vi "Global_Izleme.vi"() -> ()   [LabVIEW 2014]
uses:
  CustomControls/TSE_Status.ctl
  CustomControls/Program_States.ctl
  SharedVariables/TSE_Variables.vi
panel:
  in  "stop":bool
  out "TSE Status":T1={"Return Code"=0, "Message"="", "error in (no error)"={"status"=FALSE, "code"=0, "source"=""}, "Program State"=enum."Ön Yükleme Tamam", "Test A. Suresi"=0}
  out "GPIB_Interface_No":string
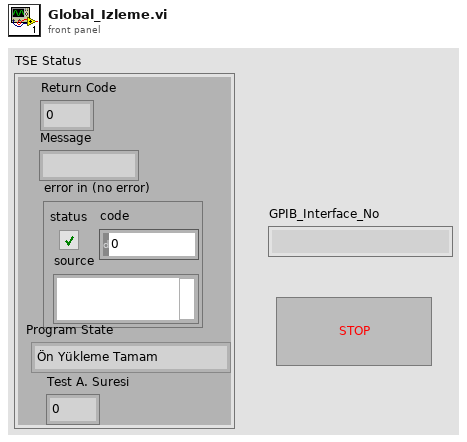
[diagram p1: front panel]
types:
  T1 = typedef "TSE_Status.ctl" = cluster{"Return Code":i32, "Message":string, "error in (no error)":errorcluster, "Program State":T2, "Test A. Suresi":u32}
  T2 = typedef "Program_States.ctl" = enum16{"Ön Yükleme", "TSE Baslat", "Kalibratöre Baglan", "Kalibratörü Baslat", "Ön Yükleme Tamam", "Frekans Testi", "Gerilim Testi", "Akim Testi", "Aktif Guc Testi", "Reaktif Guc Testi", "AC Akim Harmonik Testi", "AC Gerilim Harmonik Testi", "Flicker Testi", "Rapor Cikarma", "Yeniden Başlat", "Bekleme", "Durdur"}
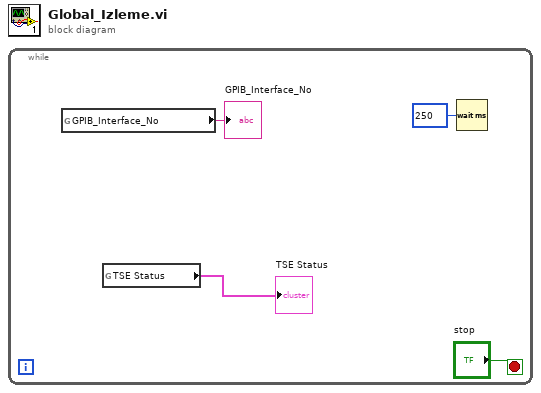
[diagram p0: block diagram]
diagram:
  n1 = while {
    stop <- "stop" stop-if-true
    n2 = global read "TSE_Variables.vi" "GPIB_Interface_No"() -> (→"GPIB_Interface_No":string)
    n3 = global read "TSE_Variables.vi" "TSE Status"() -> (→"TSE Status":T1)
    n4 = Wait (ms)(milliseconds to wait=u32 250) -> ()  [unwired: 1 out]
  }
